vi "close.vi"(8 "error in (no error)":errorcluster, 11 "hardware in":refnum<class "hardware.lvclass">) -> (0 "error out":errorcluster, 3 "hardware out":refnum<class "hardware.lvclass">)   [LabVIEW 2025, in "hardware.lvclass"]
uses:
  hardware.lvclass
  hardware.lvclass/hardware.ctl
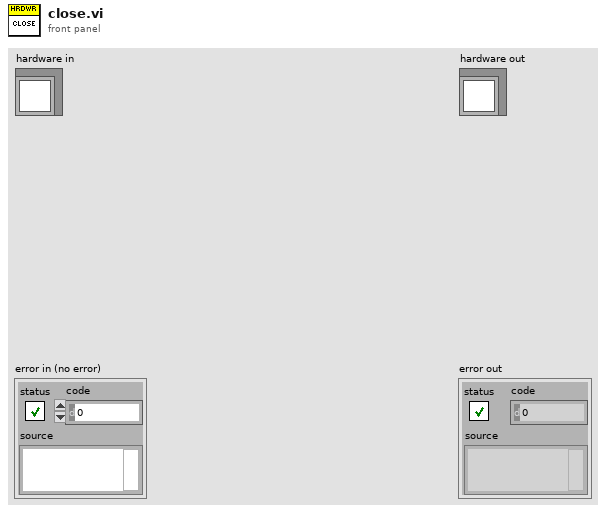
[diagram p1: front panel]
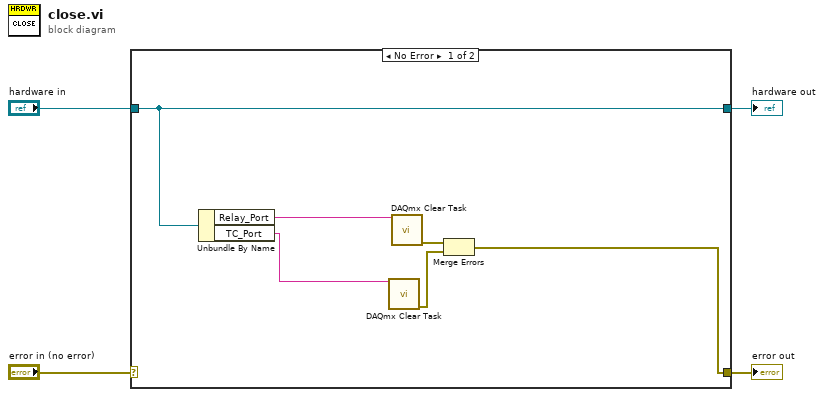
[diagram p0: block diagram]
diagram:
  n1 = case shown="No Error" "error in (no error)" {
    selector: "error in (no error)" -> [_ w12]
    tunnel: [w5 w12] -> w3
    tunnel: [w10 w11] -> w1
    tunnel: "hardware in" -> [w10 w11]
    frame No Error {
      n2 = Unbundle By Name(w10) -> ("Relay_Port"=w7:string, "TC_Port"=w6:string)
      n3 = call <vilib>:"DAQmx Clear Task.vi"("task in"=w6) -> ("error out"=w8:errorcluster)  [unwired: 14 in]
      n4 = call <vilib>:"DAQmx Clear Task.vi"("task in"=w7) -> ("error out"=w9:errorcluster)  [unwired: 14 in]
      n5 = Merge Errors(w9, w8) -> (w5:errorcluster)
    }
    frame Error {
    }
  }
  "error out" <- w3
  "hardware out" <- w1
